vi "Auto Gear Align.vi"(8 "Error In":errorcluster, 11 "Refnum's In":T1={"Gyro"="Gyro", "Mtr 1"="LeftMtr", "Mtr 2"="RightMtr"}) -> (0 "Error Out":errorcluster, 3 "Refnum's Out":T1={"Gyro"="Gyro", "Mtr 1"="LeftMtr", "Mtr 2"="RightMtr"})   [LabVIEW 2016]
uses:
  Robot Global Data.vi
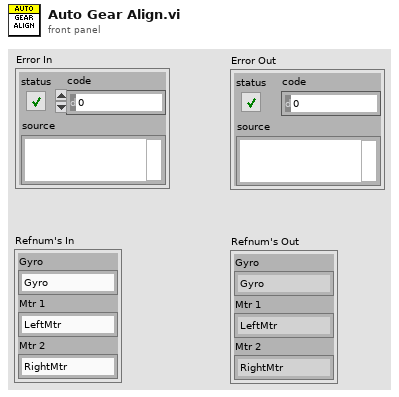
[diagram p1: front panel]
types:
  T1 = cluster{"Gyro":string, "Mtr 1":string, "Mtr 2":string}
  T2 = cluster{"Bounding Box Final":cluster{"Left":dbl, "Top":dbl, "Right":dbl, "Bottom":dbl}, "X Resolution":i32, "Y Resolution":i32}
  T3 = cluster{"Left":dbl, "Top":dbl, "Right":dbl, "Bottom":dbl}
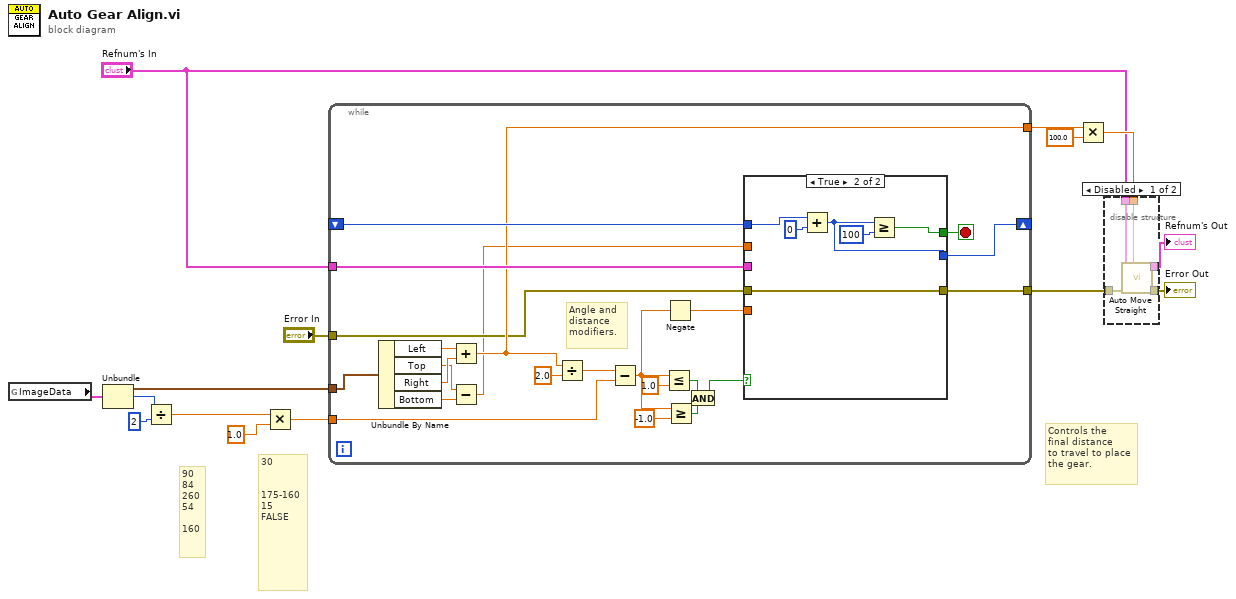
[diagram p0: block diagram]
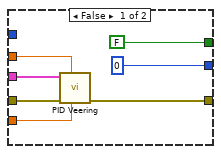
[diagram p3: hidden frame]
diagram:
  # "30\n\n\n175-160\n15\nFALSE"
  # "90\n84\n260\n54\n\n160"
  # "Controls the \nfinal distance\nto travel to place\nthe gear."
  n1 = global read "Robot Global Data.vi" "ImageData"() -> (w7:T2)
  n2 = Unbundle(w7) -> ("Bounding Box Final"=w6:T3, "X Resolution"=w4:i32)  [unwired: 1 out]
  n3 = Divide(x=w4, y=2) -> (x/y=w2:dbl)
  n4 = Multiply(x=w2, y=1.0) -> (x*y=w1:dbl)
  n5 = while {
    tunnel: "Refnum's In" -> [w35]
    shift-right: [w32] -> _
    shift-left: _ -> [w31]
    tunnel: [w30] -> w15
    tunnel: "Error In" -> [w29]
    tunnel: [w28] -> w10
    tunnel: w6 -> [w20]
    tunnel: w1 -> [w19]
    stop <- w25 stop-if-true
    # "Angle and \ndistance\nmodifiers."
    n6 = Unbundle By Name(w20) -> ("Left"=w38:dbl, "Top"=w27:dbl, "Right"=w37:dbl, "Bottom"=w26:dbl)
    n7 = Add(x=w38, y=w37) -> (x+y=w30:dbl)
    n8 = Subtract(x=w27, y=w26) -> (x-y=w16:dbl)
    n9 = Divide(x=w30, y=2.0) -> (x/y=w34:dbl)
    n10 = Subtract(x=w34, y=w19) -> (x-y=w17:dbl)
    n11 = Less Or Equal?(x=w17, y=1.0) -> (x <= y?=w23:bool)
    n12 = Negate(x=w17) -> (-x=w18:dbl)
    n13 = Greater Or Equal?(x=w17, y=-1.0) -> (x >= y?=w22:bool)
    n14 = And(x=w23, y=w22) -> (x .and. y?=w21:bool)
    n15 = case shown="True" w21 {
      tunnel: w35 -> [w42 _]
      tunnel: w18 -> [w40 _]
      tunnel: [0 w51] -> w32
      tunnel: w31 -> [_ w50]
      tunnel: [FALSE w49] -> w25
      tunnel: w29 -> [w41 w48]
      tunnel: [w39 w48] -> w28
      tunnel: w16 -> [w43 _]
      frame False {
        n16 = call "PID Veering.vi"("Error"=w40, "Current Distance"=w43, "error in (no error)"=w41, "Refnum's"=w42) -> ("error out"=w39:errorcluster)  [unwired: 7 in]
      }
      frame True {
        n17 = Add(x=w50, y=0) -> (x+y=w51:i32)
        n18 = Greater Or Equal?(x=w51, y=100) -> (x >= y?=w49:bool)
      }
    }
  }
  n19 = Multiply(x=w15, y=100.0) -> (x*y=w13:dbl)
  n20 = disable-structure shown="Disabled" {
    disable-tunnel: w13 -> [w56 _]
    disable-tunnel: [w55 _] -> w11
    disable-tunnel: w10 -> [w54 _]
    disable-tunnel: [w53 _] -> w9
    disable-tunnel: "Refnum's In" -> [w52 _]
    frame Disabled {
      n21 = call "Auto Move Straight.vi"("Target Distance"=w56, "Error In"=w54, "Refnum's In"=w52) -> ("Error Out"=w55:errorcluster, "Refnum's Out"=w53:T1)  [unwired: 7 in]
    }
    frame Enabled {
    }
  }
  "Error Out" <- w11
  "Refnum's Out" <- w9
